vi "Histogram.vi"() -> ()   [LabVIEW 2014]
doc: "This example shows how to compute the histogram of an image or a region in the image. This example also shows how to set up and use the display tools to select and work on different regions in the image interactively."
uses:
  <vilib>/vision/NI_Vision_Development_Module.lvlib
panel:
  out "Mean":sgl format="%#.2f"
  out "Standard Deviation":sgl format="%#.2f"
  out "Image":T1(plugin-control)
  out "Histogram":T2(graph)
  in  "Stop":bool
  # "Overview: Demonstrates how to use the IMAQ Histogram function with a mask to return histogram information about the portion of the image in a Region of Interest (ROI).\nRequirements: Vision Development Software.\nInstructions:\n1. Run the VI.\n2. Draw a ROI in the image by left clicking, hold left mouse button down, drag the mouse across the image, and release the mouse button."
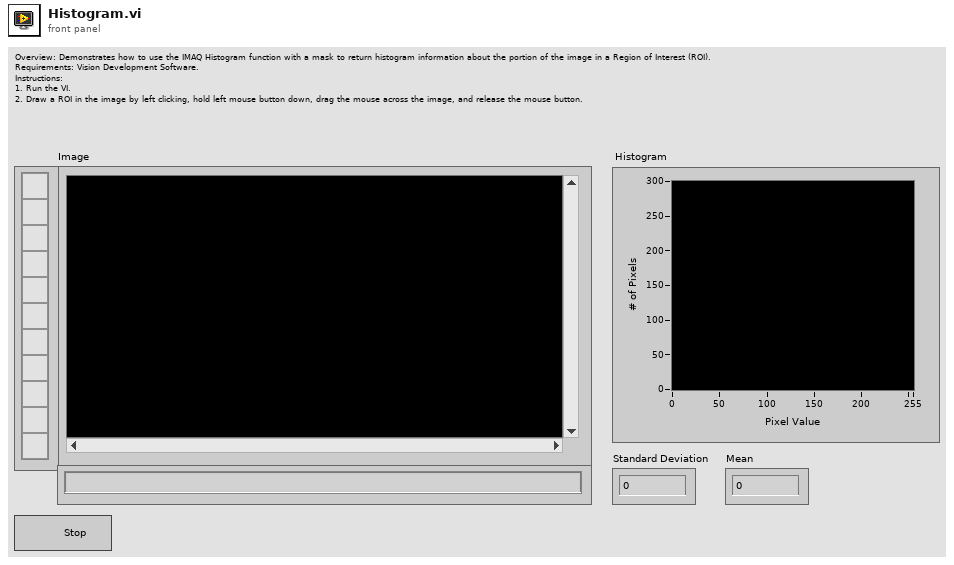
[diagram p1: front panel]
types:
  T1 = typedef "IMAQ Image.ctl" = refnum<image>
  T2 = cluster{"Starting Value":sgl, "Incremental Value":sgl, "Histogram":u32[]}
  T3 = typedef "IMAQ Rectangle" = cluster{"Left":i32, "Top":i32, "Right":i32, "Bottom":i32, "Rotation":dbl}
  T4 = typedef "ROI Descriptor" = cluster{"Global Rectangle":i32[], "Contours":cluster{"ID":enum32{"External", "Internal"}, "Type":u32, "Coordinates":i32[]}[]}
  T5 = cluster{"Global Rectangle":i32[], "Contours":cluster{"Contour Type":u32, "ROI Type":u32, "Points":i32[]}[]}
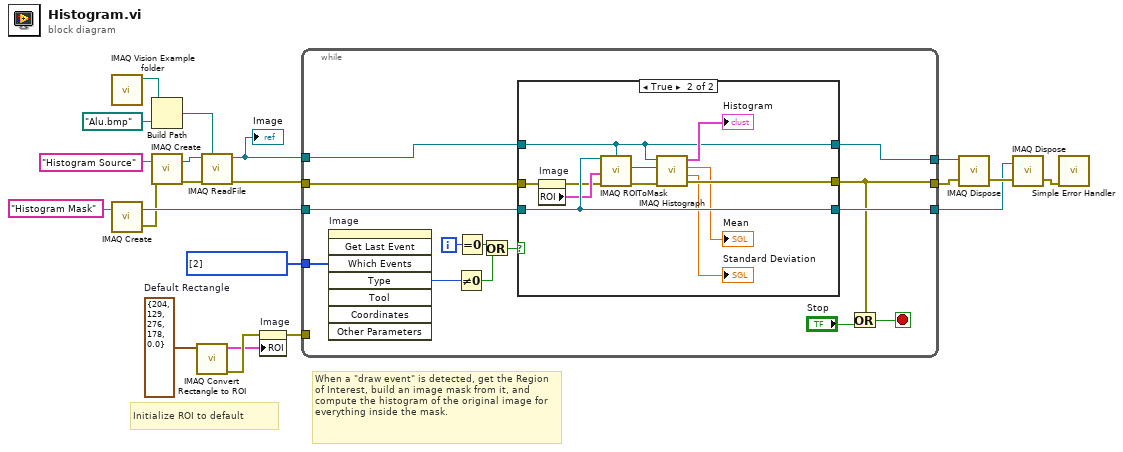
[diagram p0: block diagram]
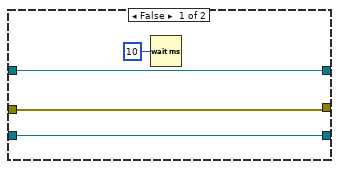
[diagram p2: hidden frame]
diagram:
  w7 = T3 {"Left"=204, "Top"=129, "Right"=276, "Bottom"=178, "Rotation"=0.0}  # Default Rectangle
  w11 = i32[] [2] items=["No  event", "Click event", "Draw event", "Move event", "Size event", "Scroll event", "Activate event", "Close event", "Double click event"] ("Events list (all)")
  # "Initialize ROI to default"
  # "When a \"draw event\" is detected, get the Region of Interest, build an image mask from it, and compute the histogram of the original image for everything inside the mask."
  n1 = call "IMAQ Vision Example folder.vi"() -> ("Example Image Path"=w21:path)  [unwired: 11 in]
  n2 = call "IMAQ Create"("Image Name"="Histogram Mask") -> ("New Image"=w15:T1, "error out"=w3:errorcluster)  [unwired: 4 in]
  n3 = Build Path(base path=w21, name or relative path=path "Alu.bmp") -> (appended path=w5:path)
  n4 = call "IMAQ Create"("Image Name"="Histogram Source", "error in (no error)"=w3) -> ("New Image"=w20:T1, "error out"=w19:errorcluster)  [unwired: 3 in]
  n5 = call "IMAQ Convert Rectangle to ROI"("Rectangle"=w7) -> ("error out"=w4:errorcluster, "ROI Descriptor"=w2:T4)  [unwired: 8 in]
  n6 = call "IMAQ ReadFile"("File Path"=w5, "error in (no error)"=w19, "Image"=w20) -> ("error out"=w17:errorcluster, "Image Out"=w8:T1)  [unwired: 4 in, 3 out]
  "Image" <- w8
  n7 = property on="Image" class="ImageControl"(error in=w4, "ROI"=w2) -> (error out=w1:errorcluster)  [unwired: 1 in, 1 out]
  n8 = while {
    tunnel: w8 -> [w29]
    tunnel: w17 -> [w30]
    tunnel: w15 -> [w31]
    tunnel: [w26] -> w14
    tunnel: [w34] -> w9
    tunnel: [w33] -> w10
    tunnel: w11 -> [w28]
    tunnel: w1 -> [_]
    i -> [w23]
    stop <- w32 stop-if-true
    n9 = invoke on="Image" class="ImageControl" method="Get Last Event"("Which Events"=w28) -> ("Type"=w27:i32)  [unwired: 7 in, 7 out]
    n10 = Not Equal To 0?(x=w27) -> (x != 0?=w25:bool)
    n11 = Equal To 0?(x=w23) -> (x = 0?=w22:bool)
    n12 = Or(x=w22, y=w25) -> (x .or. y?=w24:bool)
    n13 = case shown="True" w24 {
      tunnel: w29 -> [w38 w45]
      tunnel: w31 -> [w37 w46]
      tunnel: [w36 w48] -> w26
      tunnel: [w37 w46] -> w34
      tunnel: [w38 w45] -> w33
      tunnel: w30 -> [w36 w44]
      frame False {
        n14 = Wait (ms)(milliseconds to wait=u32 10) -> ()  [unwired: 1 out]
      }
      frame True {
        n15 = property on="Image" class="ImageControl"(error in=w44) -> (error out=w42:errorcluster, "ROI"=w43:T5)  [unwired: 1 in, 1 out]
        n16 = call "IMAQ ROIToMask"("error in (no error)"=w42, "ROI Descriptor"=w43, "Image"=w46, "Image Model"=w45) -> ("error out"=w49:errorcluster, "Image Out"=w50:T1)  [unwired: 2 in, 1 out]
        n17 = call "IMAQ Histograph"("error in (no error)"=w49, "Image Mask"=w50, "Image"=w45) -> ("error out"=w48:errorcluster, "Standard  Deviation"=→"Standard Deviation":sgl, "Mean Value"=→"Mean":sgl, "Histogram Graph"=→"Histogram":T2)  [unwired: 5 in]
      }
    }
    n18 = Or(x=w26, y="Stop") -> (x .or. y?=w32:bool)
  }
  n19 = call "IMAQ Dispose"("Image"=w10, "error in (no error)"=w14) -> ("error out"=w13:errorcluster)  [unwired: 4 in]
  n20 = call "IMAQ Dispose"("Image"=w9, "error in (no error)"=w13) -> ("error out"=w12:errorcluster)  [unwired: 4 in]
  n21 = call <vilib>:"Simple Error Handler.vi"("error in (no error)"=w12) -> ()  [unwired: 4 in, 5 out]
